vi "Enqueue (Single).vi"(4 "timeout in ms (-1)":i32=-1, 6 "Priority Message? Array":bool, 8 "error in (no error)":errorcluster, 9 "Message Data Array":variant, 10 "States":T2=enum."Default", 11 "Message Queue":T1) -> (0 "error out":errorcluster, 3 "Message Queue dub":T1)   [LabVIEW 2019, in "Acquire Mouse.lvlib"]
doc: "For a regular message, enqueue the message. For a priority message, enqueue it at the front of the queue."
uses:
  Acquire Mouse.lvlib
  State Name.ctl
  Shared/TypeDefs/Message Queue Ref.ctl
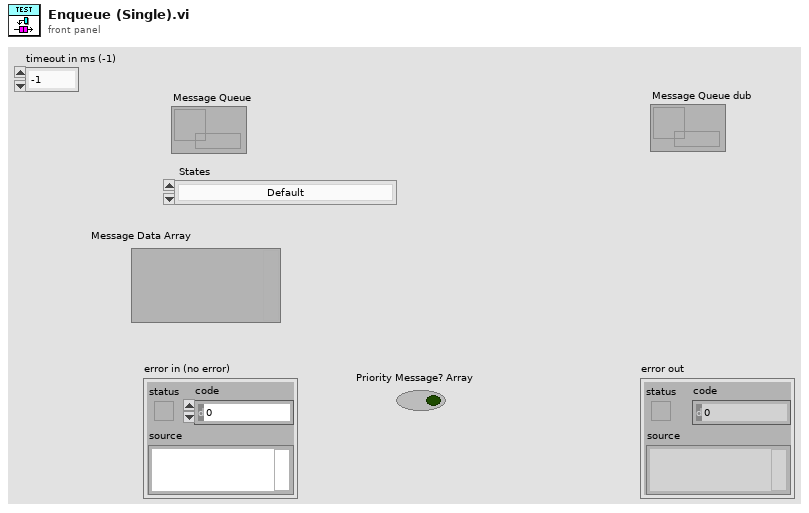
[diagram p1: front panel]
types:
  T1 = typedef "Message Queue Ref.ctl" = refnum<queue>
  T2 = typedef "Acquire Mouse.lvlib/State Name.ctl" = enum16{"Initialize", "Re-Initialize", "Initialize Data", "Initialize Panel", "[Event Structure] Update Data", "Add VI", "Get Splitters", "Map Splitter Pos to Coords", "Initialize Mouse", "Acquire Data", "Process Data", "Error", "Exit", "Default"}
  T3 = cluster{string, "Variant":variant, "call chain":string[], "Message Data Array":variant}
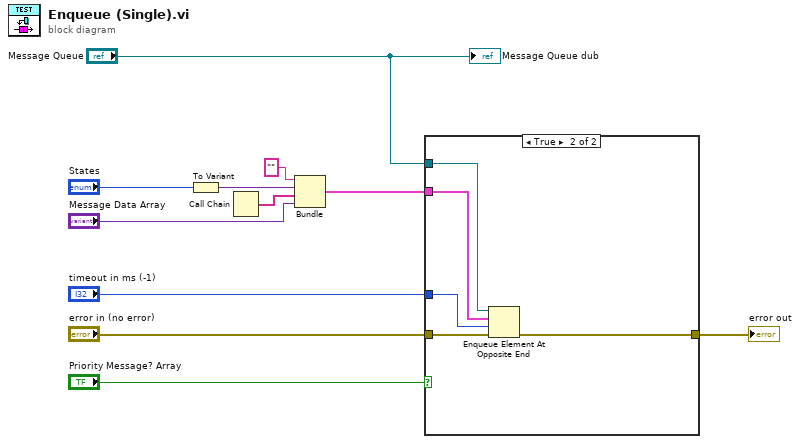
[diagram p0: block diagram]
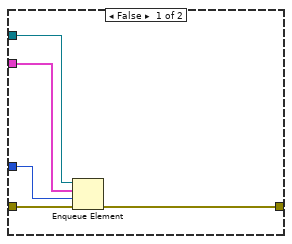
[diagram p2: hidden frame]
diagram:
  n1 = To Variant(anything="States") -> (Variant=w6:variant)
  n2 = Call Chain() -> (call chain=w4:string[])
  n3 = Bundle("", "Variant"=w6, "call chain"=w4, "Message Data Array"="Message Data Array") -> (w2:T3)  [unwired: 1 in]
  n4 = case shown="True" "Priority Message? Array" {
    tunnel: "error in (no error)" -> [w16 w21]
    tunnel: [w15 w20] -> w9
    tunnel: "Message Queue" -> [w14 w19]
    tunnel: w2 -> [w13 w18]
    tunnel: "timeout in ms (-1)" -> [w12 w17]
    frame False {
      n5 = Enqueue Element(queue=w14, element=w13, timeout in ms (-1)=w12, error in (no error)=w16) -> (error out=w15:errorcluster)  [unwired: 2 out]
    }
    frame True {
      n6 = Enqueue Element At Opposite End(queue=w19, element=w18, timeout in ms (-1)=w17, error in (no error)=w21) -> (error out=w20:errorcluster)  [unwired: 2 out]
    }
  }
  "error out" <- w9
  "Message Queue dub" <- "Message Queue"
